vi "Sample Code.vi"() -> ()   [LabVIEW 2019]
panel:
  out "Numeric":dbl
  in  "Var 2":dbl
  in  "Var 1":dbl
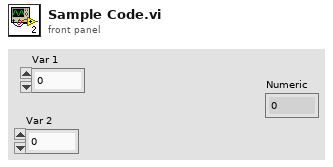
[diagram p1: front panel]
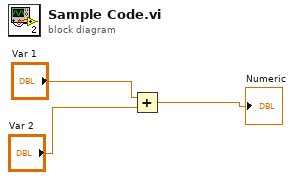
[diagram p0: block diagram]
diagram:
  n1 = Add(x="Var 1", y="Var 2") -> (x+y=→"Numeric":dbl)
